vi "Array Multipyly and Add (SubVI).vi"(10 "Array 2":i16[](array[numeric])=[0, 0, 0, 0, 0, 0, 0], 11 "Array":i16[](array[numeric])=[0, 0, 0, 0, 0, 0, 0]) -> (3 "Numeric":i32)   [LabVIEW 2017]
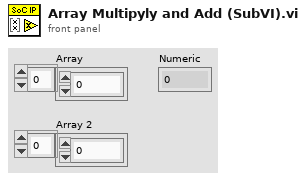
[diagram p1: front panel]
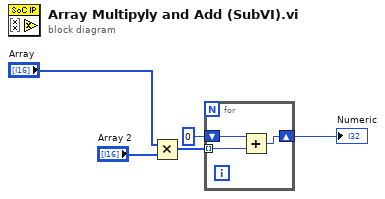
[diagram p0: block diagram]
diagram:
  n1 = Multiply(x="Array", y="Array 2") -> (x*y=w2:i32[])
  n2 = for {
    tunnel: w2 -> [w8] mode=indexing
    shift-right: [w7] -> w4
    shift-left: 0 -> [w6]
    n3 = Add(x=w6, y=w8) -> (x+y=w7:i32)
  }
  "Numeric" <- w4
